vi "set direction of axes.vi"(8 "error in":errorcluster, 9 "stage to move (def: fine)":enum16{"fine", "coarse"}(ring), 10 "direction (def: forward)":enum16{"forward", "reverse"}(ring), 11 "GPIB # (in): def. 6":string="6") -> (0 "error out":errorcluster, 3 "GPIB # (out)":string="6")   [LabVIEW 2017]
doc: "This tells the translation stage to go to the position that has previously been set."
uses:
  mc2mc4.llb/MC2/4  SendCommand.VI
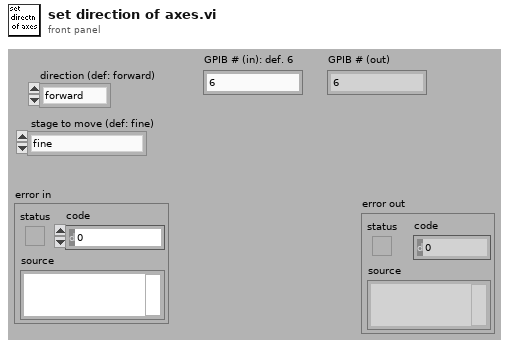
[diagram p1: front panel]
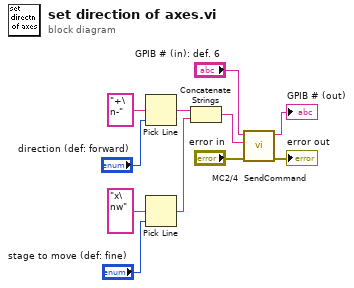
[diagram p0: block diagram]
diagram:
  n1 = Pick Line(multi-line string="+\n-", line index="direction (def: forward)") -> (output string=w5:string)  [unwired: 1 out]
  n2 = Pick Line(multi-line string="x\nw", line index="stage to move (def: fine)") -> (output string=w4:string)  [unwired: 1 out]
  n3 = Concatenate Strings(w5, w4) -> (w3:string)
  n4 = call "MC2/4  SendCommand.VI"("error in (no error)"="error in", "MC2 / MC4 Command"=w3, "GPIB # (in): def.6"="GPIB # (in): def. 6") -> ("error out"=→"error out":errorcluster, "GPIB # (out)"=→"GPIB # (out)":string)  [unwired: 7 out]
